vi "UI Cycle Filter.vi"(10 "filter?":bool, 11 "Menu in":refnum<k9>) -> ()   [LabVIEW 2012]
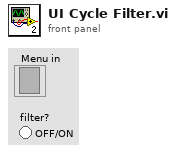
[diagram p1: front panel]
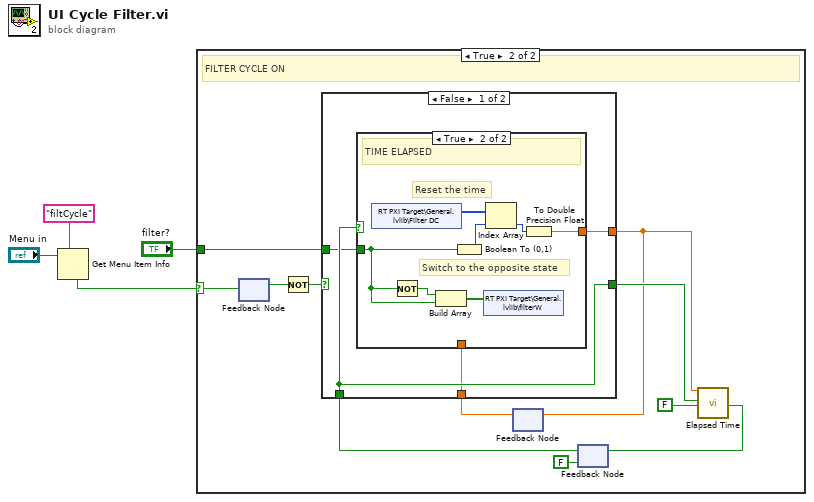
[diagram p0: block diagram]
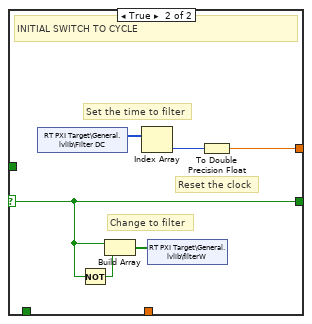
[diagram p4: hidden frame]
diagram:
  n1 = Get Menu Item Info(7:"filtCycle" ("item tag"), 11:"Menu in") -> (4:w3:bool)  [unwired: 1 in, 6 out]
  n2 = case shown="True" w3 {
    selector: w3 -> [_ w15]
    tunnel: "filter?" -> [_ w6]
    frame False {
    }
    frame True {
      # "FILTER CYCLE ON"
      n3 = feedback-in #1(w15) -> ()
      n4 = feedback #1() -> (w14:bool)  [unwired: 1 in]
      n5 = Not(x=w14) -> (.not. x?=w13:bool)
      n6 = feedback #2() -> (w7:dbl)  [unwired: 1 in]
      n7 = feedback #3(FALSE ("Time has Elapsed")) -> (w9:bool)
      n8 = case shown="False" w13 {
        selector: w13 -> [_ w32]
        tunnel: [w19 w32] -> w12
        tunnel: w9 -> [w19 _]
        tunnel: [w18 w28] -> w8
        tunnel: w7 -> [w17 _]
        tunnel: w6 -> [w16 _]
        frame False {
          n9 = case shown="True" w19 {
            tunnel: [w20 w24] -> w18
            tunnel: w17 -> [w20 _]
            tunnel: w16 -> [_ w21]
            frame False {
              # "TIME NOT ELAPSED"
            }
            frame True {
              # "Switch to the opposite state"
              # "Reset the time"
              # "TIME ELAPSED"
              n10 = shared-variable "RT PXI Target\\General.lvlib\\Filter DC"() -> (w27:u16[])  [unwired: 1 in, 1 out]
              n11 = Not(x=w21) -> (.not. x?=w23:bool)
              n12 = Build Array(w23, w21) -> (w22:bool[])
              n13 = Boolean To (0,1)(Boolean=w21) -> (0, 1=w26:i16)
              n14 = shared-variable "RT PXI Target\\General.lvlib\\filterW"(w22) -> ()  [unwired: 1 in, 1 out]
              n15 = Index Array(array=w27, index=w26) -> (element=w25:u16)
              n16 = To Double Precision Float(number=w25) -> (double precision float=w24:dbl)
            }
          }
        }
        frame True {
          # "Set the time to filter"
          # "Change to filter"
          # "Reset the clock"
          # "INITIAL SWITCH TO CYCLE"
          n17 = shared-variable "RT PXI Target\\General.lvlib\\Filter DC"() -> (w30:u16[])  [unwired: 1 in, 1 out]
          n18 = Not(x=w32) -> (.not. x?=w33:bool)
          n19 = Build Array(w32, w33) -> (w31:bool[])
          n20 = Index Array(array=w30) -> (element=w29:u16)  [unwired: 1 in]
          n21 = shared-variable "RT PXI Target\\General.lvlib\\filterW"(w31) -> ()  [unwired: 1 in, 1 out]
          n22 = To Double Precision Float(number=w29) -> (double precision float=w28:dbl)
        }
      }
      n23 = feedback-in #2(w8) -> ()
      n24 = call "Elapsed Time"("Time Target (s)"=w8, "Reset"=w12, "Auto Reset"=FALSE) -> ("Time has Elapsed"=w10:bool)  [unwired: 9 in, 7 out]
      n25 = feedback-in #3(w10) -> ()
    }
  }
